vi "calculated Lower Fault.vi"(8 "error in (no error)":errorcluster, 10 "Input Values":sgl[](array[numeric]), 11 "AILimitConfig":T1(array[cluster])) -> (0 "error out":errorcluster, 2 "LF Events":string[](array[string]), 3 "LF Channel":string[](array[string]))   [LabVIEW 2018]
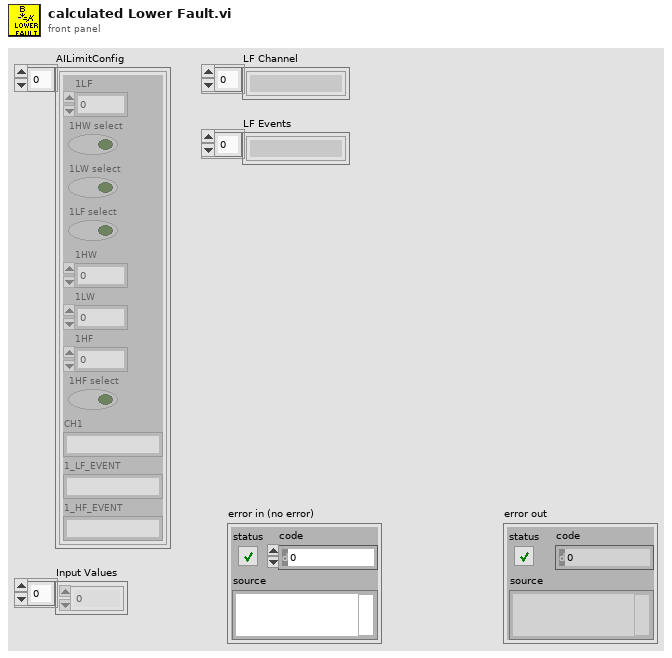
[diagram p1: front panel]
types:
  T1 = cluster{"1LF":dbl, "1HW select":bool, "1LW select":bool, "1LF select":bool, "1HW":dbl, "1LW":dbl, "1HF":dbl, "1HF select":bool, "CH1":string, "1_LF_EVENT":string, "1_HF_EVENT":string}[]
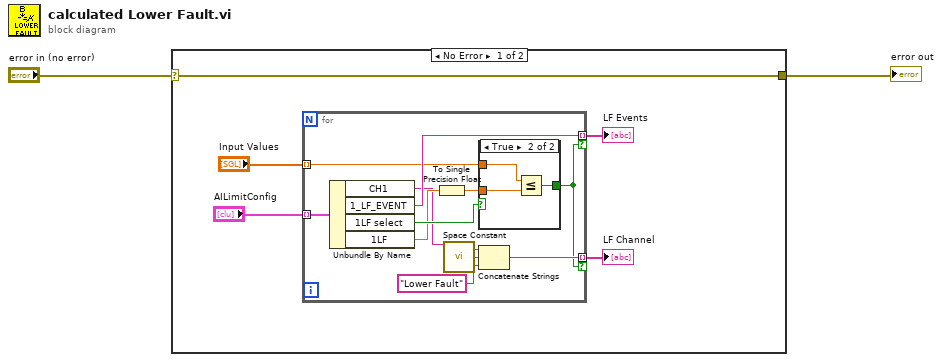
[diagram p0: block diagram]
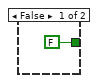
[diagram p2: hidden frame]
diagram:
  n1 = case shown="No Error" "error in (no error)" {
    selector: "error in (no error)" -> [w3 w23]
    tunnel: [w3 w23] -> w1
    frame No Error {
      n2 = for {
        tunnel: "AILimitConfig" -> [w18] mode=indexing
        tunnel: [w17] -> w6 mode=indexing if=w9
        tunnel: "Input Values" -> [w14] mode=indexing
        tunnel: [w10] -> w5 mode=indexing if=w9
        n3 = Unbundle By Name(w18) -> ("CH1"=w11:string, "1_LF_EVENT"=w17:string, "1LF select"=w16:bool, "1LF"=w15:dbl)
        n4 = To Single Precision Float(number=w15) -> (single precision float=w8:sgl)
        n5 = call <vilib>:"Space Constant.vi"() -> ("String"=w13:string)
        n6 = case shown="True" w16 {
          tunnel: w14 -> [_ w22]
          tunnel: w8 -> [_ w21]
          tunnel: [FALSE w20] -> w9
          frame False {
          }
          frame True {
            n7 = Less Or Equal?(x=w22, y=w21) -> (x <= y?=w20:bool)
          }
        }
        n8 = Concatenate Strings(w11, w13, "Lower Fault" ("string")) -> (w10:string)
      }
      "LF Events" <- w6
      "LF Channel" <- w5
    }
    frame Error {
    }
  }
  "error out" <- w1
